vi "Analyzer.vi"(6 "采样点数":i32, 7 "分析方法":enum16{"过零法", "相关法", "FFT频谱分析法"}(ring), 8 "采样频率":dbl, 9 "信号频率":dbl, 10 "波形 2":dbl[](graph), 11 "波形 1":dbl[](graph)) -> (3 "相位差":dbl)   [LabVIEW 2022 SP3]
uses:
  <vilib>/Analysis/2dsp.llb/1D Auto Correlation (DBL).vi
  <vilib>/express/express analysis/Spectral/Block/exnSpectralBlock spectral measurements peak poly.vi
  <vilib>/express/express analysis/Spectral/Block/exnSpectralBlock spectral measurements peak WFM.vi
  <vilib>/Analysis/2dsp.llb/1D Cross Correlation (DBL).vi
  <vilib>/express/express analysis/Spectral/XNode/ExpressSpectralMeasurementsBlockNode.xnode
  <vilib>/Analysis/NI_AALPro.lvlib
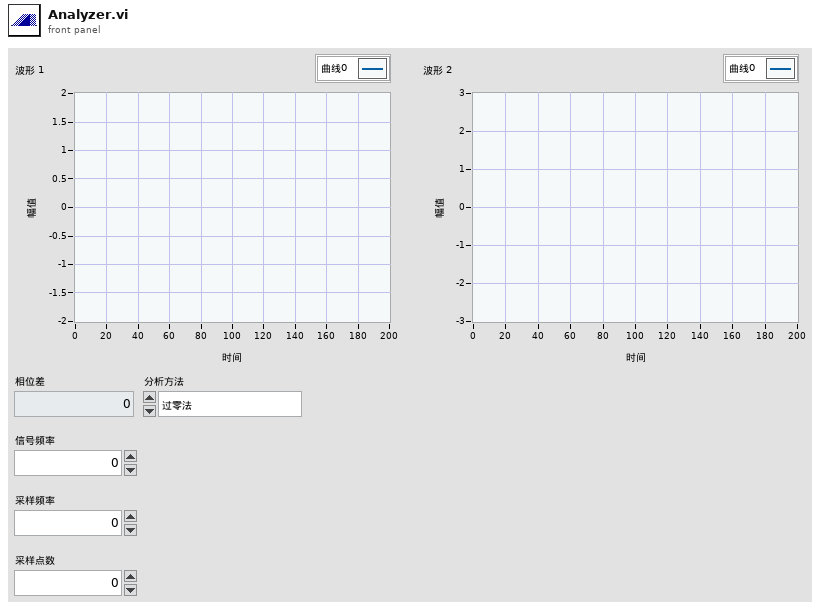
[diagram p1: front panel]
types:
  T1 = cluster{"averaging mode":u16, "weighting mode":u16, "number of averages":u32}
  T2 = cluster{"dB On (F)":bool, "unwrap phase (F)":bool, "convert to degree (F)":bool}
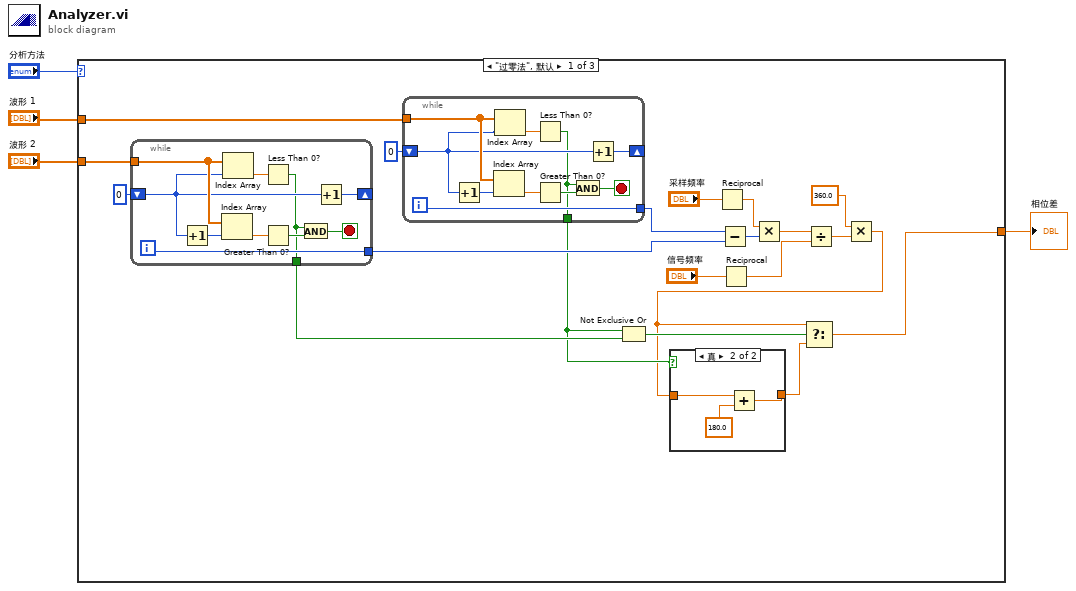
[diagram p0: block diagram]
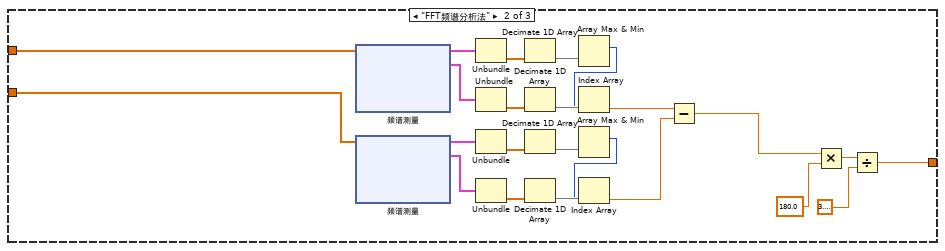
[diagram p3: hidden frame]
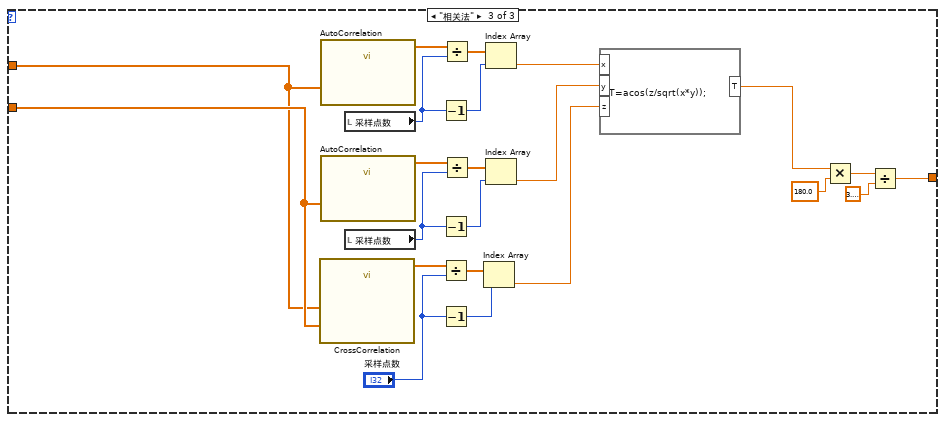
[diagram p4: hidden frame]
diagram:
  n1 = case shown="\"过零法\", 默认" "分析方法" {
    tunnel: "波形 2" -> [w23 w53 w93]
    tunnel: "波形 1" -> [w21 w54 w92]
    tunnel: [w10 w49 w94] -> w1
    frame "过零法", Default {
      n2 = while {
        shift-right: [w48] -> _
        shift-left: 0 -> [w40]
        tunnel: w23 -> [w46]
        tunnel: [w41] -> w18
        tunnel: [w39] -> w14
        i -> [w41]
        stop <- w42 stop-if-true
        n3 = Increment(x=w40) -> (x+1=w44:i32)
        n4 = Index Array(array=w46, index=w44) -> (element=w45:dbl)
        n5 = Index Array(array=w46, index=w40) -> (element=w47:dbl)
        n6 = Less Than 0?(x=w47) -> (x < 0?=w39:bool)
        n7 = Greater Than 0?(x=w45) -> (x > 0?=w43:bool)
        n8 = And(x=w39, y=w43) -> (x .and. y?=w42:bool)
        n9 = Increment(x=w40) -> (x+1=w48:i32)
      }
      n10 = while {
        shift-right: [w38] -> _
        shift-left: 0 -> [w30]
        tunnel: w21 -> [w36]
        tunnel: [w31] -> w17
        tunnel: [w29] -> w12
        i -> [w31]
        stop <- w32 stop-if-true
        n11 = Increment(x=w30) -> (x+1=w34:i32)
        n12 = Index Array(array=w36, index=w34) -> (element=w35:dbl)
        n13 = Index Array(array=w36, index=w30) -> (element=w37:dbl)
        n14 = Less Than 0?(x=w37) -> (x < 0?=w29:bool)
        n15 = Greater Than 0?(x=w35) -> (x > 0?=w33:bool)
        n16 = And(x=w29, y=w33) -> (x .and. y?=w32:bool)
        n17 = Increment(x=w30) -> (x+1=w38:i32)
      }
      n18 = Not Exclusive Or(1:w14, 2:w12) -> (0:w15:bool)
      n19 = Reciprocal(x="采样频率") -> (1/x=w8:dbl)
      n20 = Subtract(x=w17, y=w18) -> (x-y=w16:i32)
      n21 = Reciprocal(x="信号频率") -> (1/x=w5:dbl)
      n22 = Multiply(x=w8, y=w16) -> (x*y=w9:dbl)
      n23 = Divide(x=w9, y=w5) -> (x/y=w20:dbl)
      n24 = Multiply(x=360.0, y=w20) -> (x*y=w11:dbl)
      n25 = case shown="真" w12 {
        tunnel: [w25 w27] -> w13
        tunnel: w11 -> [w25 w26]
        frame False {
        }
        frame True {
          n26 = Add(x=w26, y=180.0) -> (x+y=w27:dbl)
        }
      }
      n27 = Select(t=w11, s=w15, f=w13) -> (s? t:f=w10:dbl)
    }
    frame "FFT频谱分析法" {
      n28 = xnode "频谱测量"("信号"=w54) -> ("FFT - （峰值）"=w68:cluster{"f0":dbl, "df":dbl, "magnitude":dbl[]}, "相位"=w67:cluster{"f0":dbl, "df":dbl, "phase":dbl[]})  [unwired: 1 in, 1 out]
      n29 = xnode "频谱测量"("信号"=w53) -> ("FFT - （峰值）"=w58:cluster{"f0":dbl, "df":dbl, "magnitude":dbl[]}, "相位"=w57:cluster{"f0":dbl, "df":dbl, "phase":dbl[]})  [unwired: 1 in, 1 out]
      n30 = Unbundle(w68) -> ("magnitude"=w69:dbl[])  [unwired: 2 out]
      n31 = Unbundle(w67) -> ("phase"=w66:dbl[])  [unwired: 2 out]
      n32 = Unbundle(w58) -> ("magnitude"=w59:dbl[])  [unwired: 2 out]
      n33 = Unbundle(w57) -> ("phase"=w56:dbl[])  [unwired: 2 out]
      n34 = Decimate 1D Array(w69) -> (w71:dbl[])  [unwired: 2 out]
      n35 = Decimate 1D Array(w66) -> (w70:dbl[])  [unwired: 2 out]
      n36 = Decimate 1D Array(w59) -> (w61:dbl[])  [unwired: 2 out]
      n37 = Decimate 1D Array(w56) -> (w60:dbl[])  [unwired: 2 out]
      n38 = Array Max & Min(array=w71) -> (max index (indices)=w65:i32)  [unwired: 3 out]
      n39 = Index Array(array=w70, index=w65) -> (element=w51:dbl)
      n40 = Array Max & Min(array=w61) -> (max index (indices)=w55:i32)  [unwired: 3 out]
      n41 = Index Array(array=w60, index=w55) -> (element=w50:dbl)
      n42 = Subtract(x=w51, y=w50) -> (x-y=w52:dbl)
      n43 = Multiply(x=w52, y=180.0) -> (x*y=w64:dbl)
      n44 = Divide(x=w64, y=3.141592653589793) -> (x/y=w49:dbl)
    }
    frame "相关法" {
      n45 = call-poly <vilib>:"CrossCorrelation.vi"("Y"=w93, "X"=w92) -> ("Rxy"=w109:dbl[])  [unwired: 8 in, 1 out]
      n46 = call-poly <vilib>:"AutoCorrelation.vi"("X"=w92) -> ("Rxx"=w107:dbl[])  [unwired: 9 in, 1 out]
      n47 = call-poly <vilib>:"AutoCorrelation.vi"("X"=w93) -> ("Rxx"=w98:dbl[])  [unwired: 9 in, 1 out]
      n48 = local read "采样点数"() -> (w100:i32)
      n49 = local read "采样点数"() -> (w96:i32)
      n50 = Decrement(x=w100) -> (x-1=w112:i32)
      n51 = Decrement(x=w96) -> (x-1=w97:i32)
      n52 = Divide(x=w109, y="采样点数") -> (x/y=w110:dbl[])
      n53 = Decrement(x="采样点数") -> (x-1=w111:i32)
      n54 = Divide(x=w107, y=w100) -> (x/y=w113:dbl[])
      n55 = Divide(x=w98, y=w96) -> (x/y=w99:dbl[])
      n56 = Index Array(array=w110, index=w111) -> (element=w108:dbl)
      n57 = Index Array(array=w113, index=w112) -> (element=w102:dbl)
      n58 = Index Array(array=w99, index=w97) -> (element=w95:dbl)
      n59 = formula code="T=acos(z/sqrt(x*y));"("y"=w95, "z"=w108, "x"=w102) -> ("T"=w106:dbl)
      n60 = Multiply(x=w106, y=180.0) -> (x*y=w105:dbl)
      n61 = Divide(x=w105, y=3.141592653589793) -> (x/y=w94:dbl)
    }
  }
  "相位差" <- w1
